vi "Lift Cases.vi"() -> ()   [LabVIEW 2014]
uses:
  Begin/Global Variables.vi
panel:
  in  "Lift Speed Slow idle":dbl=0.6
  in  "Lift Speed Fast":dbl=0.75
  in  "Pickup":dbl=32.0 format="%#_13g"
  in  "Tote 2 Height":dbl=24.0 format="%#_13g"
  in  "Tote 2 Height New":dbl=44.0
  in  "Tote 1 Height New":dbl=7.0
  in  "Tote 3 Height New":dbl=44.0
  in  "Tote 1 Height":dbl=7.5
  in  "Tote 3 Height":dbl=45.5
  in  "Lift Speed":dbl=0.95 format="%#_13g"
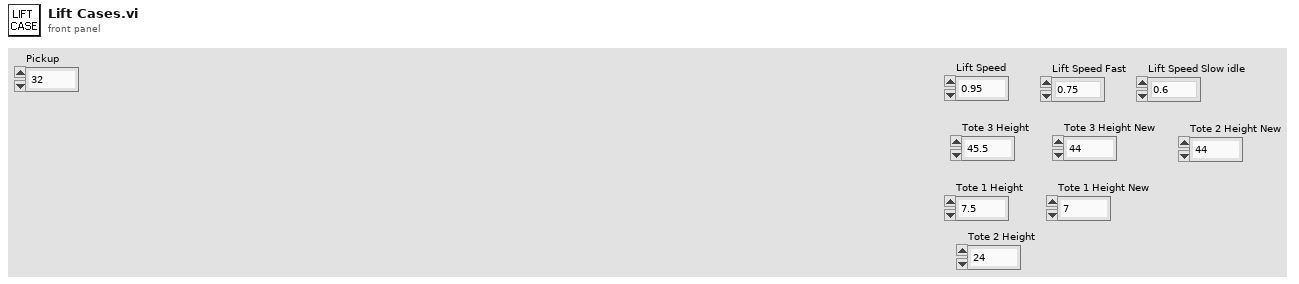
[diagram p1: front panel]
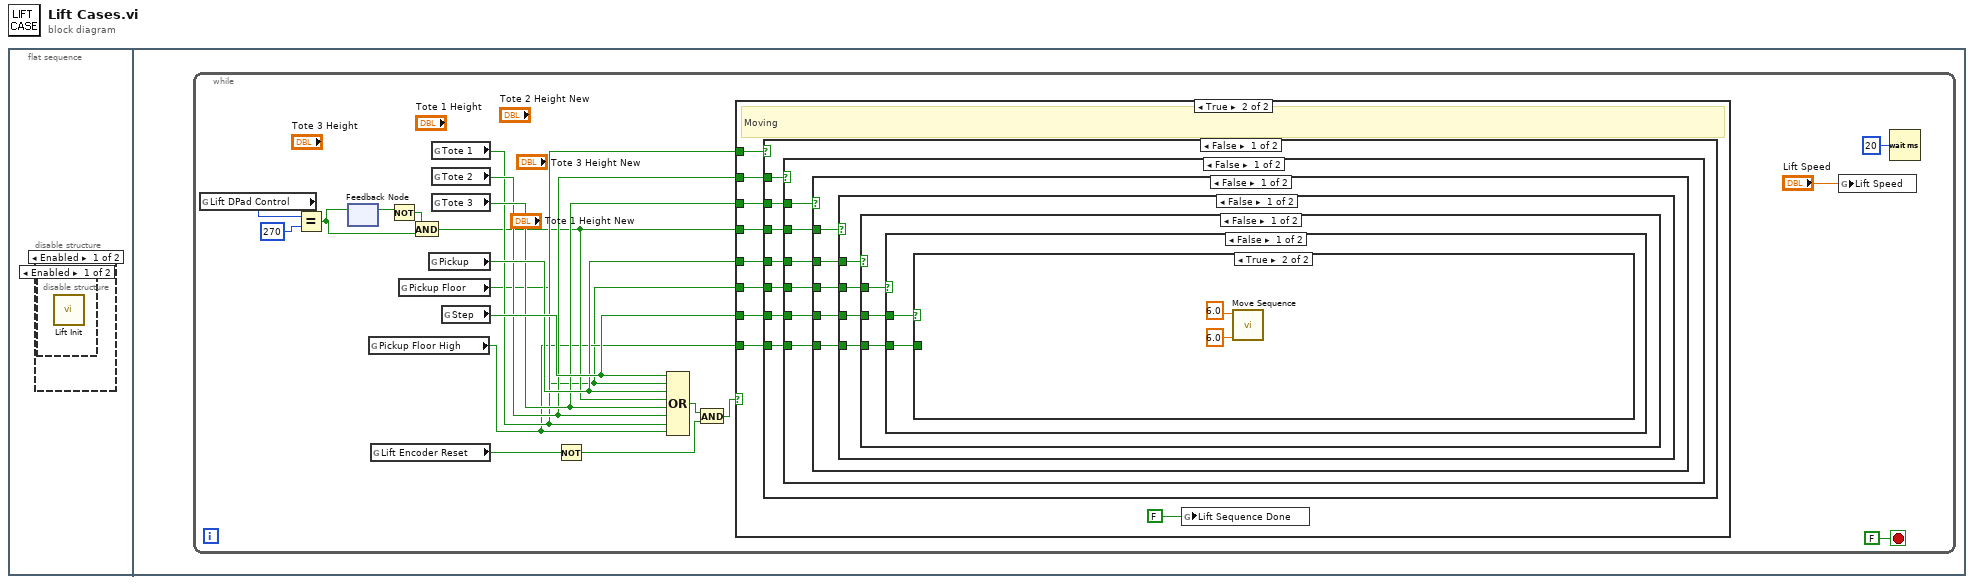
[diagram p0: block diagram]
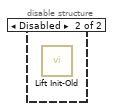
[diagram p2: hidden frame]
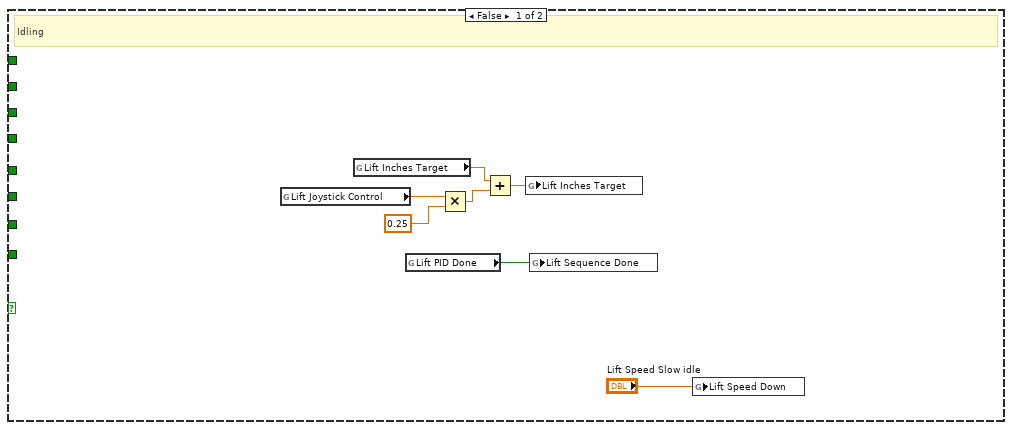
[diagram p4: hidden frame]
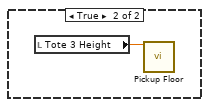
[diagram p6: hidden frame]
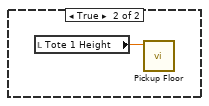
[diagram p7: hidden frame]
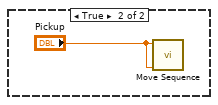
[diagram p8: hidden frame]
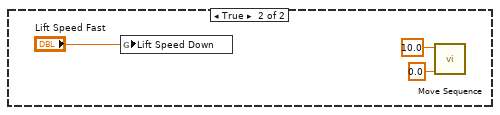
[diagram p9: hidden frame]
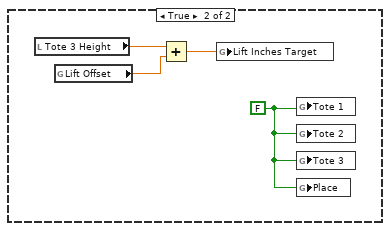
[diagram p10: hidden frame]
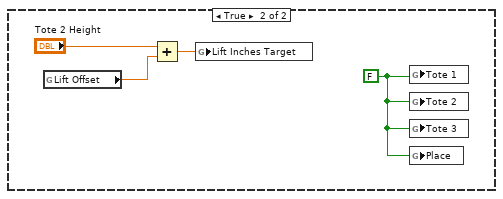
[diagram p11: hidden frame]
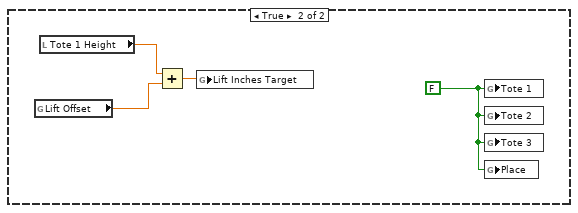
[diagram p12: hidden frame]
diagram:
  n1 = flat-sequence {
    frame #0 {
      n2 = disable-structure shown="Enabled" {
        frame Enabled {
          n3 = disable-structure shown="Enabled" {
            frame Enabled {
              n4 = call "Lift Init.vi"() -> ()  [unwired: 12 in]
            }
            frame Disabled {
              n5 = call "Lift Init-Old.vi"() -> ()  [unwired: 12 in]
            }
          }
        }
        frame Disabled {
        }
      }
    }
    frame #1 {
      n6 = while {
        stop <- FALSE stop-if-true
        n7 = global read "Global Variables.vi" "Lift DPad Control"() -> (w6:i16)
        n8 = Equal?(x=w6, y=i16 270) -> (x = y?=w11:bool)
        n9 = feedback #1() -> (w10:bool)  [unwired: 1 in]
        n10 = feedback-in #1(w11) -> ()
        n11 = global read "Global Variables.vi" "Pickup Floor High"() -> (w5:bool)
        n12 = global read "Global Variables.vi" "Lift Encoder Reset"() -> (w13:bool)
        n13 = Not(x=w10) -> (.not. x?=w9:bool)
        n14 = global read "Global Variables.vi" "Pickup Floor"() -> (w3:bool)
        n15 = And(x=w9, y=w11) -> (x .and. y?=w7:bool)
        n16 = global read "Global Variables.vi" "Pickup"() -> (w18:bool)
        n17 = global read "Global Variables.vi" "Tote 1"() -> (w15:bool)
        n18 = global read "Global Variables.vi" "Tote 2"() -> (w16:bool)
        n19 = global read "Global Variables.vi" "Tote 3"() -> (w17:bool)
        n20 = global read "Global Variables.vi" "Step"() -> (w19:bool)
        n21 = Not(x=w13) -> (.not. x?=w12:bool)
        n22 = Compound Arithmetic op=OR(w19, w3, w18, w7, w17, w16, w15, w5) -> (w2:bool)
        n23 = And(x=w2, y=w12) -> (x .and. y?=w1:bool)
        n24 = case shown="True" w1 {
          tunnel: w15 -> [_ w36]
          tunnel: w16 -> [_ w35]
          tunnel: w17 -> [_ w34]
          tunnel: w7 -> [_ w33]
          tunnel: w18 -> [_ w32]
          tunnel: w3 -> [_ w31]
          tunnel: w19 -> [_ w30]
          tunnel: w5 -> [_ w28]
          frame False {
            # "Idling"
            n25 = global read "Global Variables.vi" "Lift Joystick Control"() -> (w23:dbl)
            n26 = global read "Global Variables.vi" "Lift Inches Target"() -> (w25:dbl)
            n27 = global read "Global Variables.vi" "Lift PID Done"() -> (w27:bool)
            n28 = Multiply(x=w23, y=0.25) -> (x*y=w24:dbl)
            n29 = Add(x=w25, y=w24) -> (x+y=w26:dbl)
            n30 = global write "Global Variables.vi" "Lift Inches Target"(w26) -> ()
            n31 = global write "Global Variables.vi" "Lift Sequence Done"(w27) -> ()
            n32 = global write "Global Variables.vi" "Lift Speed Down"("Lift Speed Slow idle") -> ()
          }
          frame True {
            # "Moving"
            n33 = case shown="False" w36 {
              tunnel: w35 -> [w43 _]
              tunnel: w34 -> [w42 _]
              tunnel: w33 -> [w41 _]
              tunnel: w32 -> [w40 _]
              tunnel: w31 -> [w39 _]
              tunnel: w30 -> [w38 _]
              tunnel: w28 -> [w37 _]
              frame False {
                n34 = case shown="False" w43 {
                  tunnel: w42 -> [w49 _]
                  tunnel: w41 -> [w48 _]
                  tunnel: w40 -> [w47 _]
                  tunnel: w39 -> [w46 _]
                  tunnel: w38 -> [w45 _]
                  tunnel: w37 -> [w44 _]
                  frame False {
                    n35 = case shown="False" w49 {
                      tunnel: w48 -> [w54 _]
                      tunnel: w47 -> [w53 _]
                      tunnel: w46 -> [w52 _]
                      tunnel: w45 -> [w51 _]
                      tunnel: w44 -> [w50 _]
                      frame False {
                        n36 = case shown="False" w54 {
                          tunnel: w53 -> [w58 _]
                          tunnel: w52 -> [w57 _]
                          tunnel: w51 -> [w56 _]
                          tunnel: w50 -> [w55 _]
                          frame False {
                            n37 = case shown="False" w58 {
                              tunnel: w57 -> [w61 _]
                              tunnel: w56 -> [w60 _]
                              tunnel: w55 -> [w59 _]
                              frame False {
                                n38 = case shown="False" w61 {
                                tunnel: w60 -> [w63 _]
                                tunnel: w59 -> [w62 _]
                                frame False {
                                n39 = case shown="True" w63 {
                                tunnel: w62 -> [w64 _]
                                frame False {
                                n40 = case shown="False" w64 {
                                frame False {
                                }
                                frame True {
                                n41 = local read "Tote 3 Height"() -> (w65:dbl)
                                n42 = call "Pickup Floor.vi"("Final Height"=w65) -> ()  [unwired: 11 in]
                                }
                                }
                                }
                                frame True {
                                n43 = call "Move Sequence.vi"("Distance Up"=6.0, "Distance Down"=6.0) -> ()  [unwired: 10 in]
                                }
                                }
                                }
                                frame True {
                                n44 = local read "Tote 1 Height"() -> (w68:dbl)
                                n45 = call "Pickup Floor.vi"("Final Height"=w68) -> ()  [unwired: 11 in]
                                }
                                }
                              }
                              frame True {
                                n46 = call "Move Sequence.vi"("Distance Up"="Pickup", "Distance Down"="Pickup") -> ()  [unwired: 10 in]
                              }
                            }
                          }
                          frame True {
                            n47 = global write "Global Variables.vi" "Lift Speed Down"("Lift Speed Fast") -> ()
                            n48 = call "Move Sequence.vi"("Distance Up"=0.0, "Distance Down"=10.0 ("Distance Down 2")) -> ()  [unwired: 10 in]
                          }
                        }
                      }
                      frame True {
                        w74 = FALSE ("Tote 0")
                        n49 = local read "Tote 3 Height"() -> (w73:dbl)
                        n50 = global read "Global Variables.vi" "Lift Offset"() -> (w75:dbl)
                        n51 = Add(x=w73, y=w75) -> (x+y=w76:dbl)
                        n52 = global write "Global Variables.vi" "Lift Inches Target"(w76) -> ()
                        n53 = global write "Global Variables.vi" "Tote 1"(w74) -> ()
                        n54 = global write "Global Variables.vi" "Tote 2"(w74) -> ()
                        n55 = global write "Global Variables.vi" "Tote 3"(w74) -> ()
                        n56 = global write "Global Variables.vi" "Place"(w74) -> ()
                      }
                    }
                  }
                  frame True {
                    w77 = FALSE ("Tote 0")
                    n57 = global read "Global Variables.vi" "Lift Offset"() -> (w78:dbl)
                    n58 = Add(x="Tote 2 Height", y=w78) -> (x+y=w79:dbl)
                    n59 = global write "Global Variables.vi" "Lift Inches Target"(w79) -> ()
                    n60 = global write "Global Variables.vi" "Tote 1"(w77) -> ()
                    n61 = global write "Global Variables.vi" "Tote 2"(w77) -> ()
                    n62 = global write "Global Variables.vi" "Tote 3"(w77) -> ()
                    n63 = global write "Global Variables.vi" "Place"(w77) -> ()
                  }
                }
              }
              frame True {
                w82 = FALSE ("Tote 0")
                n64 = global read "Global Variables.vi" "Lift Offset"() -> (w83:dbl)
                n65 = local read "Tote 1 Height"() -> (w81:dbl)
                n66 = Add(x=w81, y=w83) -> (x+y=w84:dbl)
                n67 = global write "Global Variables.vi" "Lift Inches Target"(w84) -> ()
                n68 = global write "Global Variables.vi" "Tote 1"(w82) -> ()
                n69 = global write "Global Variables.vi" "Tote 2"(w82) -> ()
                n70 = global write "Global Variables.vi" "Tote 3"(w82) -> ()
                n71 = global write "Global Variables.vi" "Place"(w82) -> ()
              }
            }
            n72 = global write "Global Variables.vi" "Lift Sequence Done"(FALSE ("Lift Sequence Done")) -> ()
          }
        }
        n73 = global write "Global Variables.vi" "Lift Speed"("Lift Speed") -> ()
        n74 = Wait (ms)(milliseconds to wait=u32 20) -> ()  [unwired: 1 out]
      }
    }
  }
